vi "ORS_DatafileClose.vi"(8 "error in":errorcluster, 11 "file refnum":refnum<file>) -> (0 "error out":errorcluster)   [LabVIEW 2021]
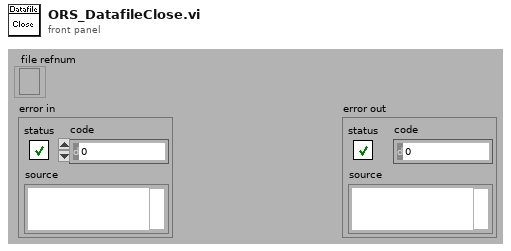
[diagram p1: front panel]
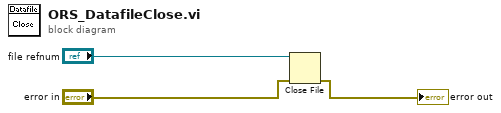
[diagram p0: block diagram]
diagram:
  n1 = Close File(refnum="file refnum", error in="error in") -> (error out=→"error out":errorcluster)  [unwired: 1 out]
